vi "Read Value.vi"(6 "Gantry in":refnum<class "Gantry.lvclass">, 8 "error in (no error)":errorcluster, 10 "String in":string, 11 "gScript Interpreter in":refnum<class "gScript Interpreter.lvclass">) -> (0 "error out":errorcluster, 2 "Memory Cell":T1, 3 "gScript Interpreter out":refnum<class "gScript Interpreter.lvclass">, 4 "Gantry out":refnum<class "Gantry.lvclass">)   [LabVIEW 2026, in "gScript Interpreter.lvclass"]
uses:
  gScript Interpreter.lvclass
  Type Definitions/Memory Cell.ctl
  Type Definitions/Memory Cell Type Enum.ctl
  Shared Components/Gantry Class/Gantry.lvclass
  <vilib>/ErrorRing/Error Ring.xnode
  <vilib>/regexp/Match Regular Expression.xnode
  Shared Components/FlexWorktable/FlexWorktable.lvclass
  gScript Interpreter.lvclass/gScript Interpreter.ctl
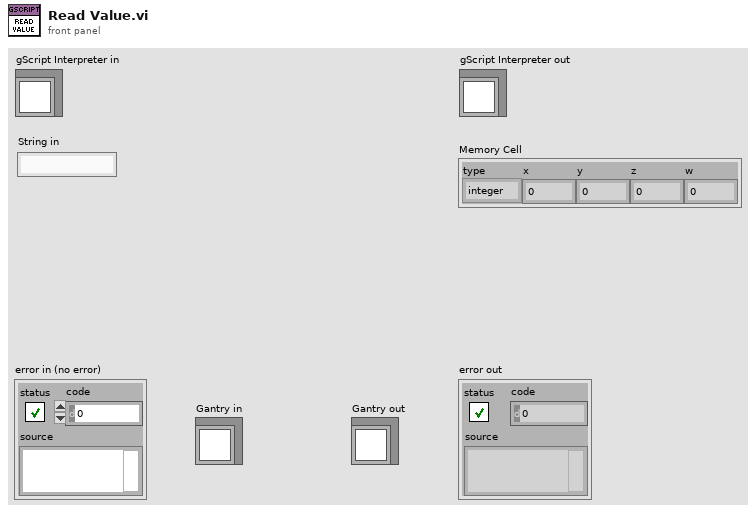
[diagram p1: front panel]
types:
  T1 = typedef "Memory Cell.ctl" = cluster{"type":T2, "x":dbl, "y":dbl, "z":dbl, "w":dbl}
  T2 = typedef "Memory Cell Type Enum.ctl" = enum16{"integer", "float", "vector", "rotation"}
  T3 = cluster{i32, dbl, string, bool, "Orient3d Class.lvclass":refnum<class "Orient3d.lvclass">, "Vec3d Class.lvclass":refnum<class "Vec3d.lvclass">}
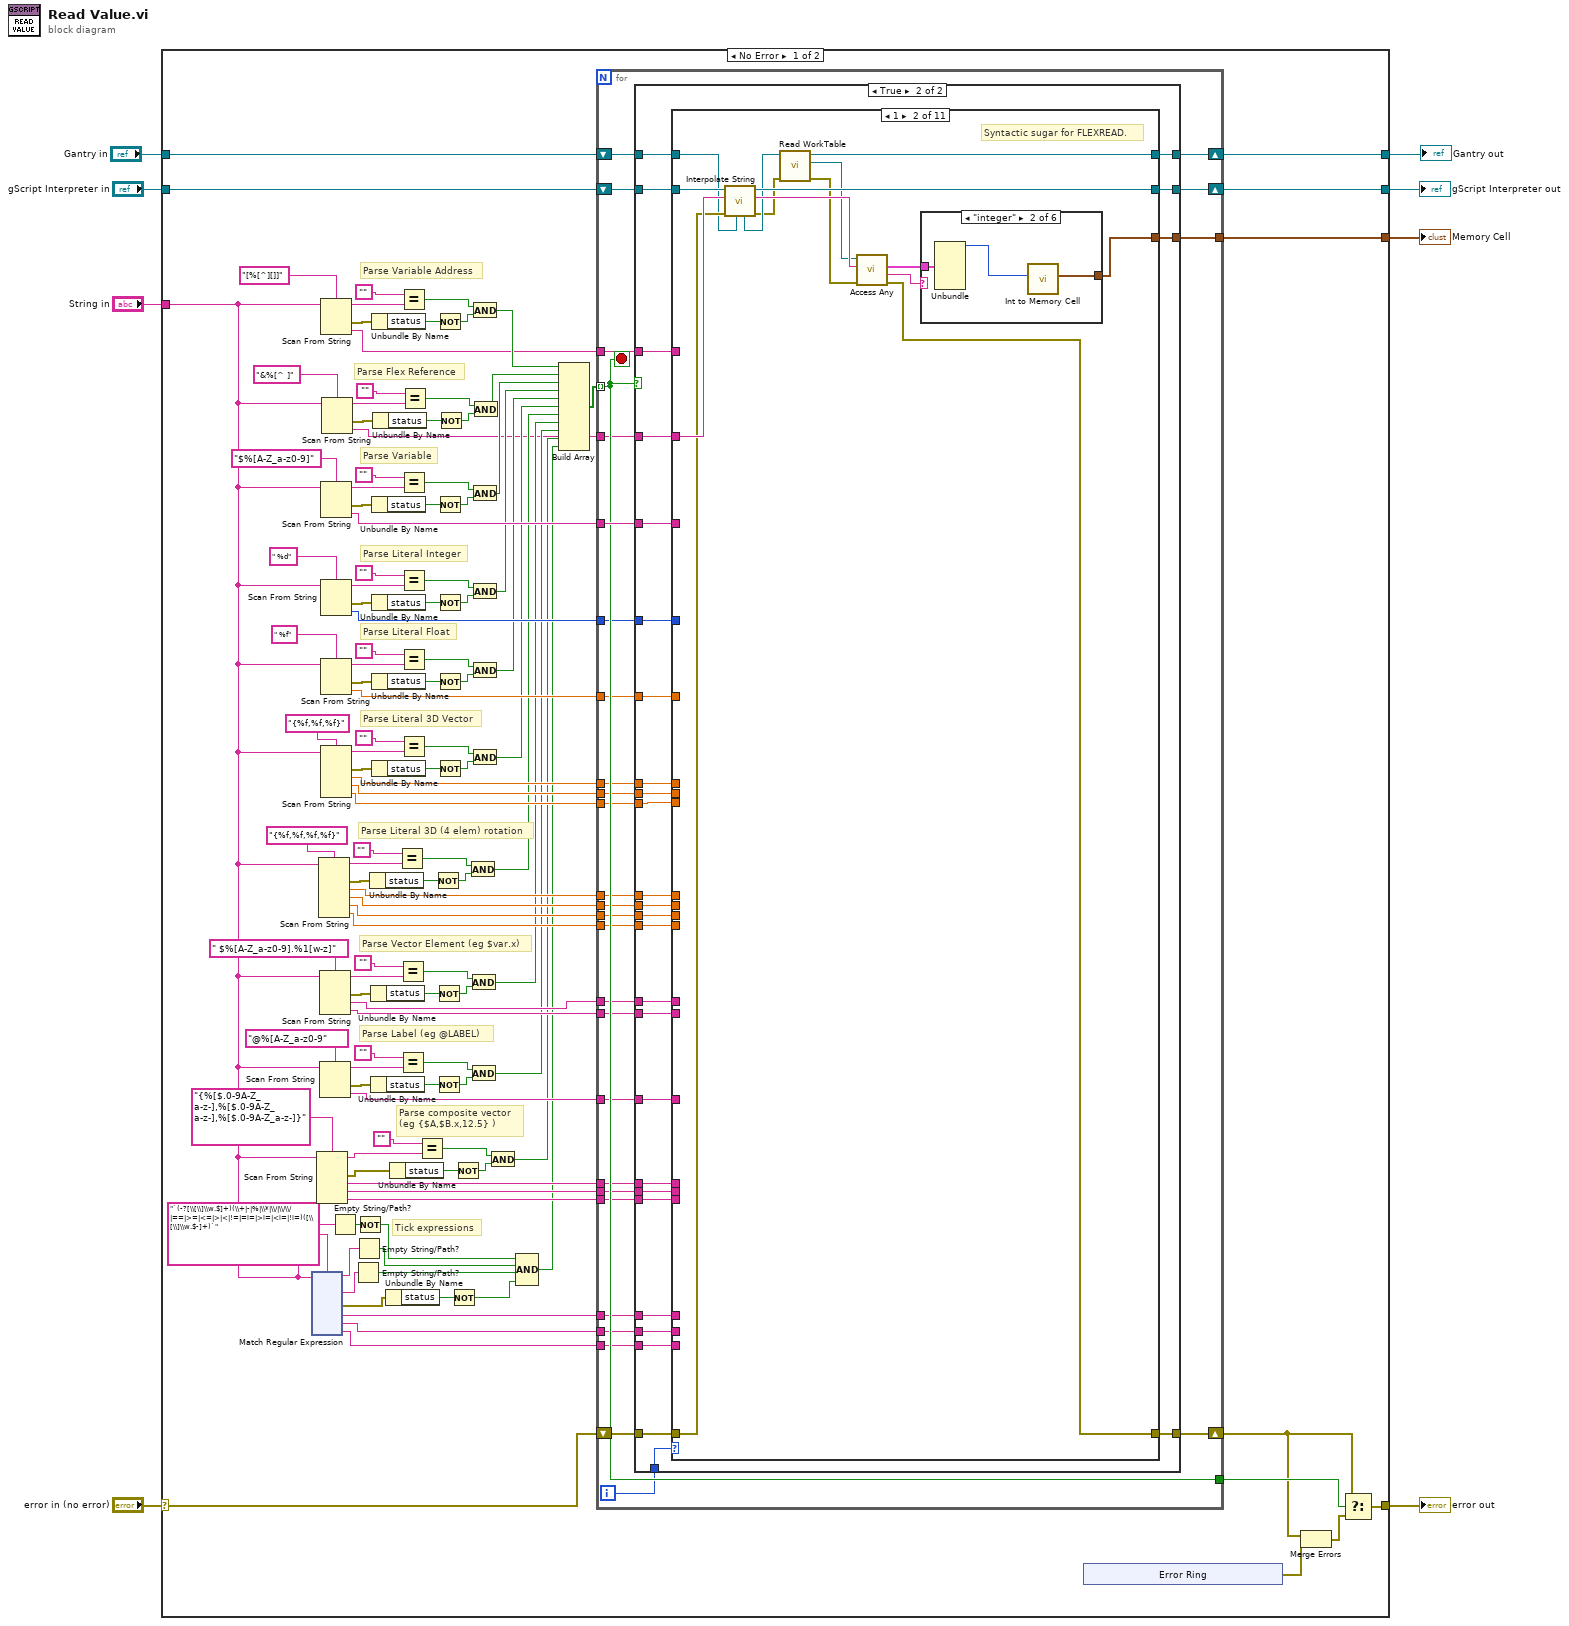
[diagram p0: block diagram]
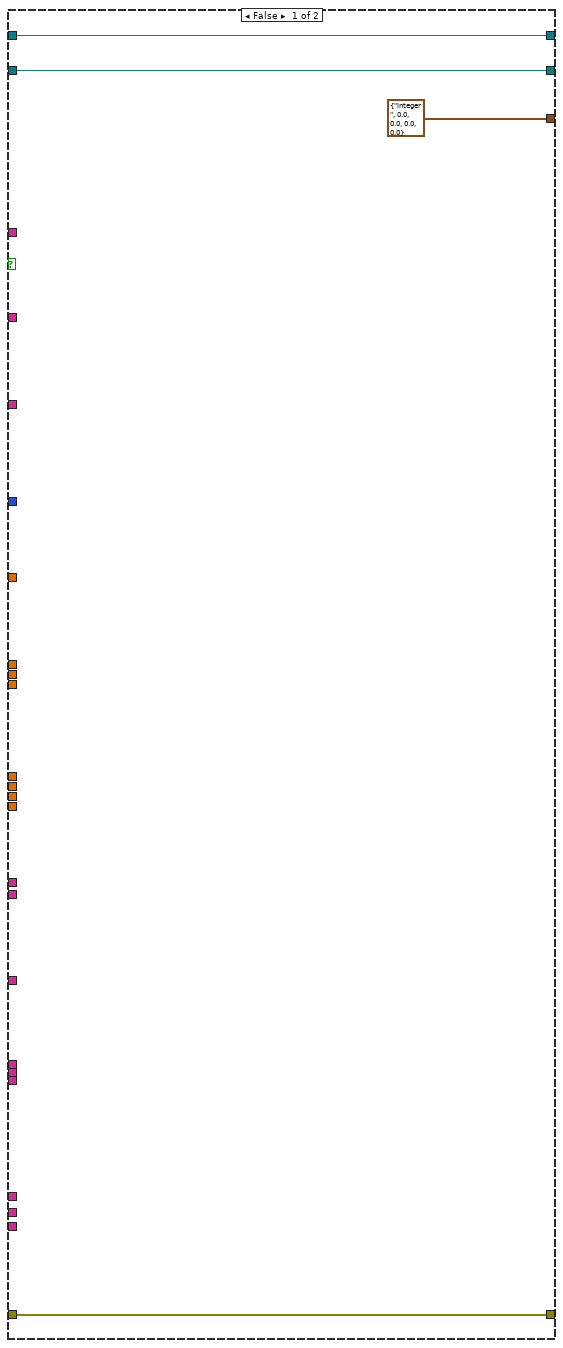
[diagram p2: hidden frame]
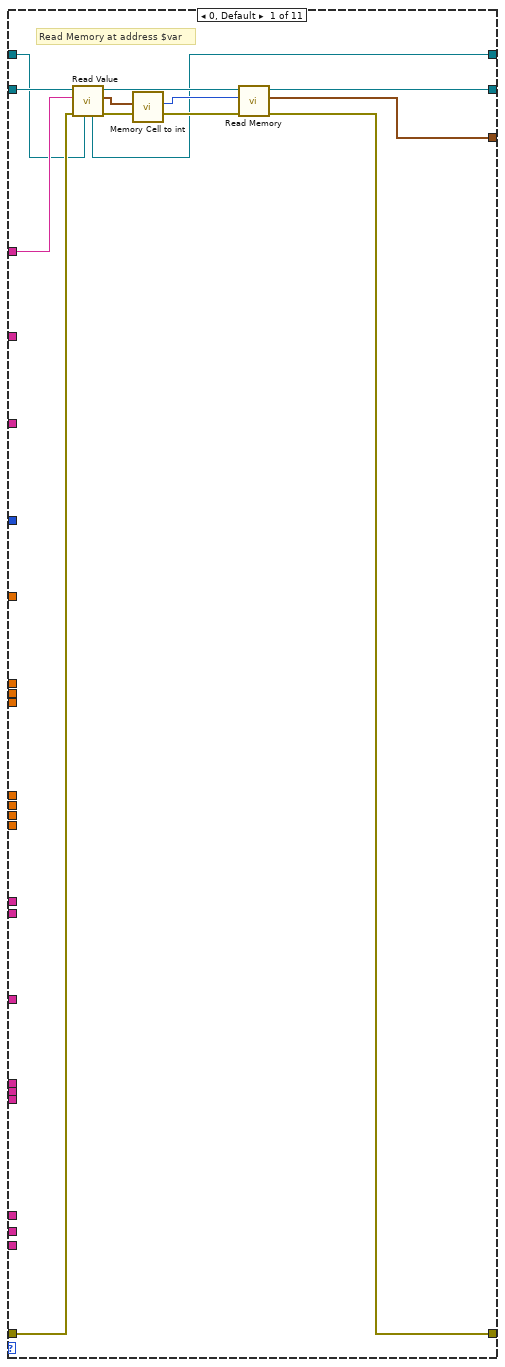
[diagram p3: hidden frame]
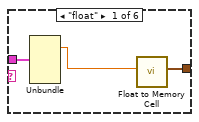
[diagram p4: hidden frame]
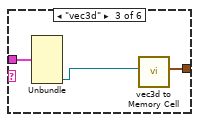
[diagram p5: hidden frame]
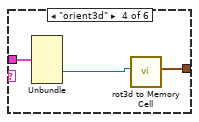
[diagram p6: hidden frame]
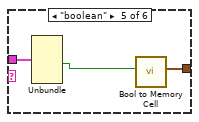
[diagram p7: hidden frame]
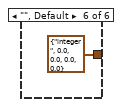
[diagram p8: hidden frame]
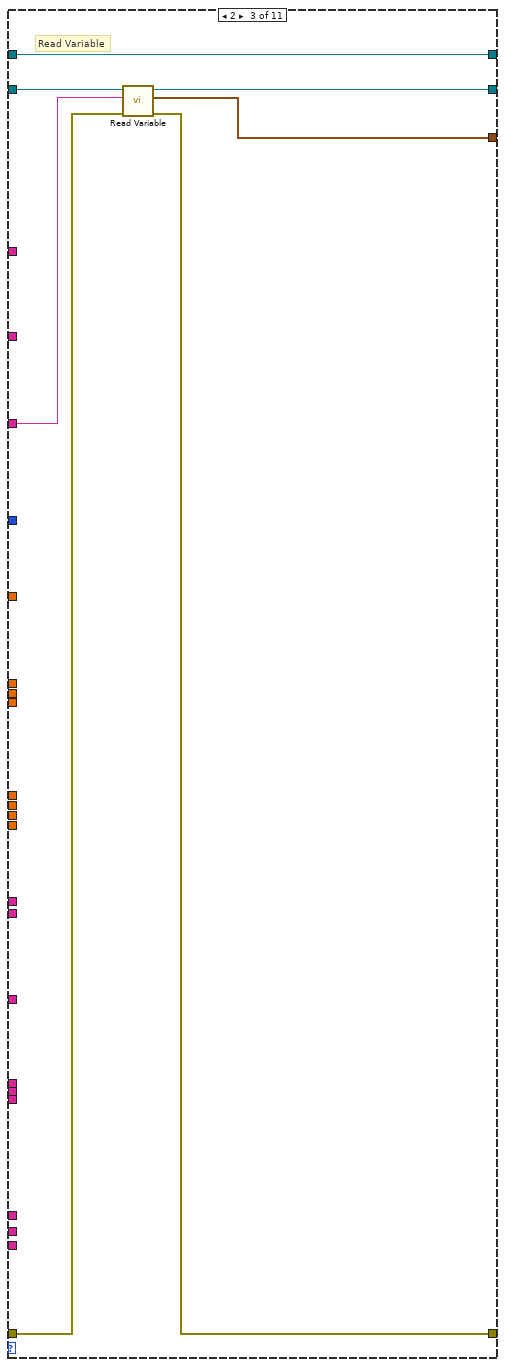
[diagram p9: hidden frame]
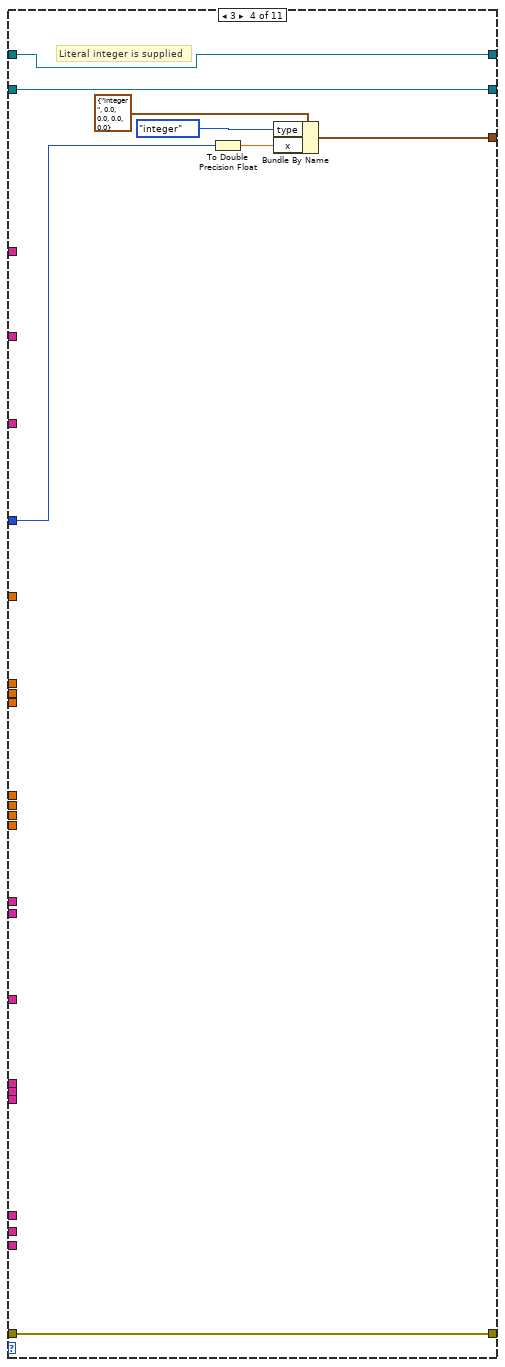
[diagram p10: hidden frame]
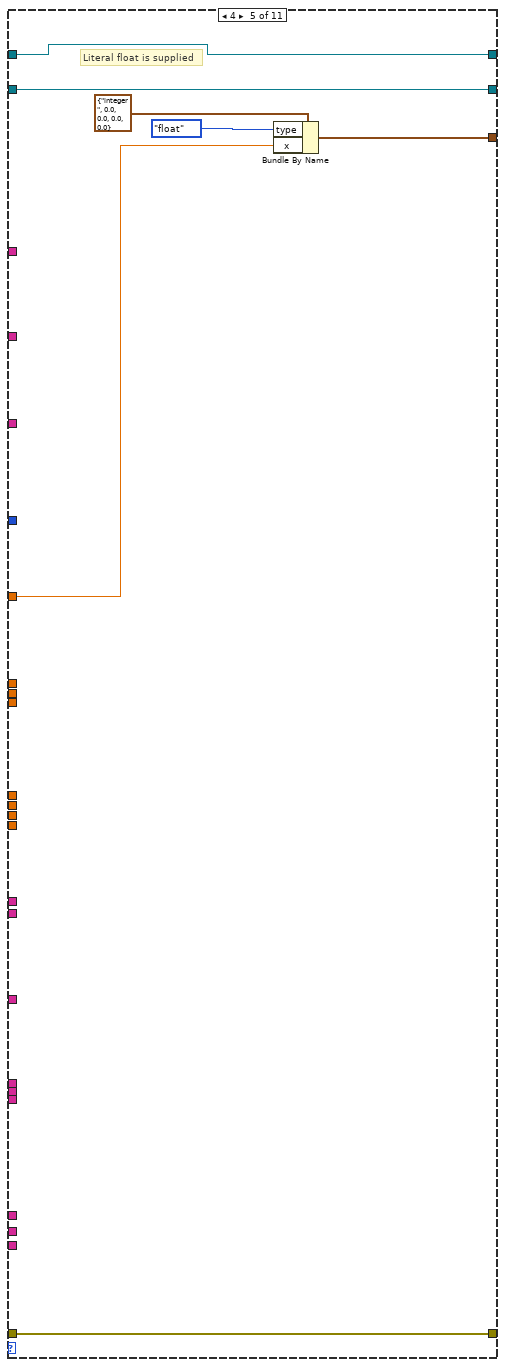
[diagram p11: hidden frame]
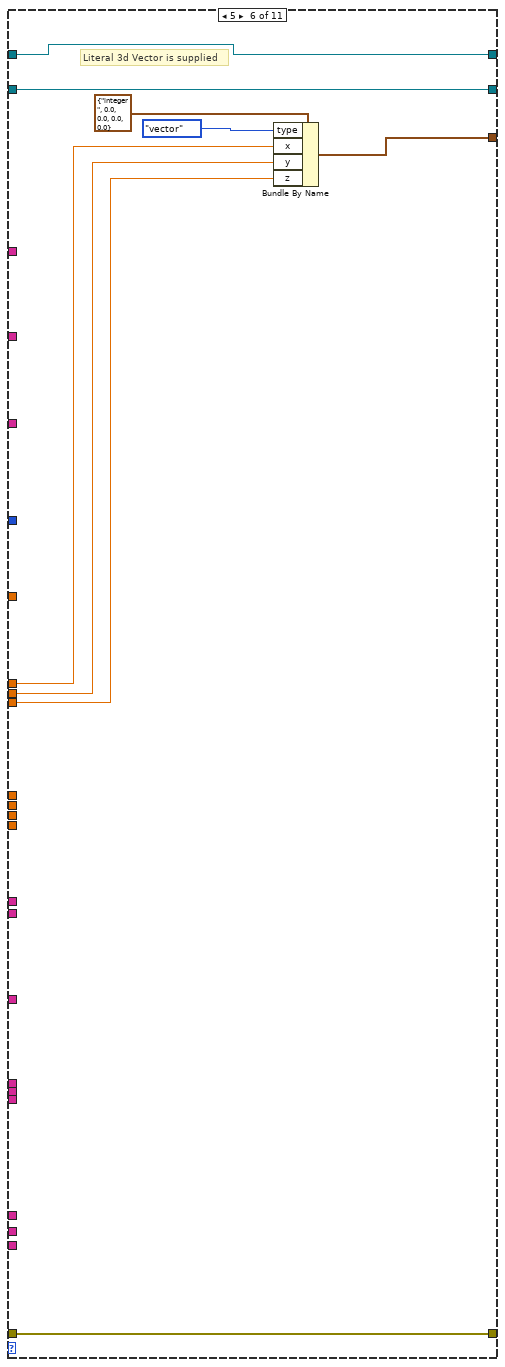
[diagram p12: hidden frame]
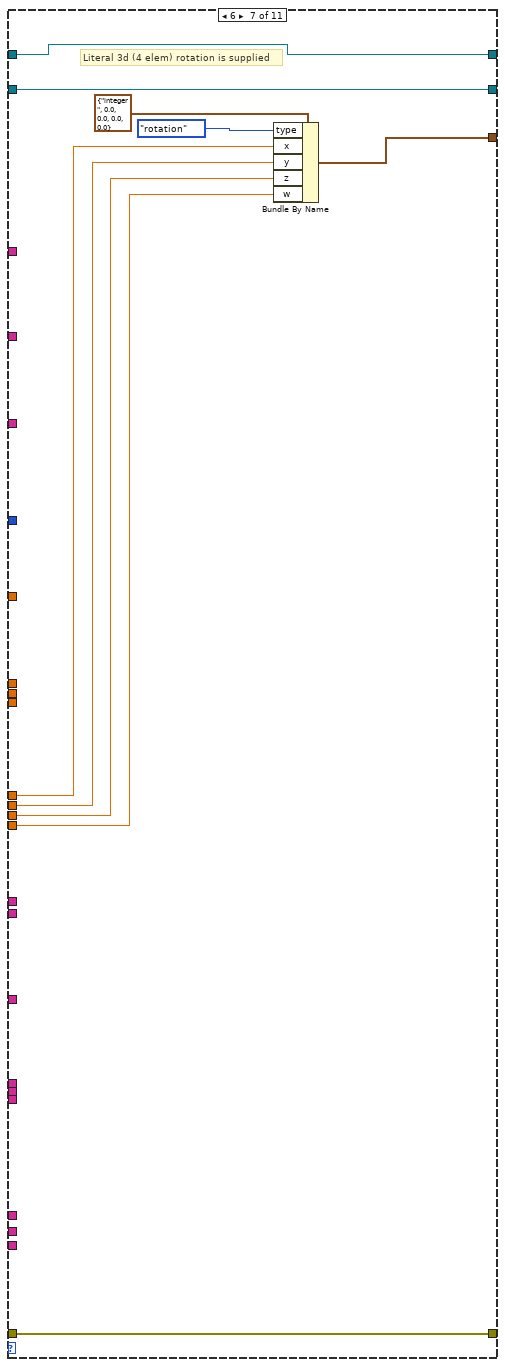
[diagram p13: hidden frame]
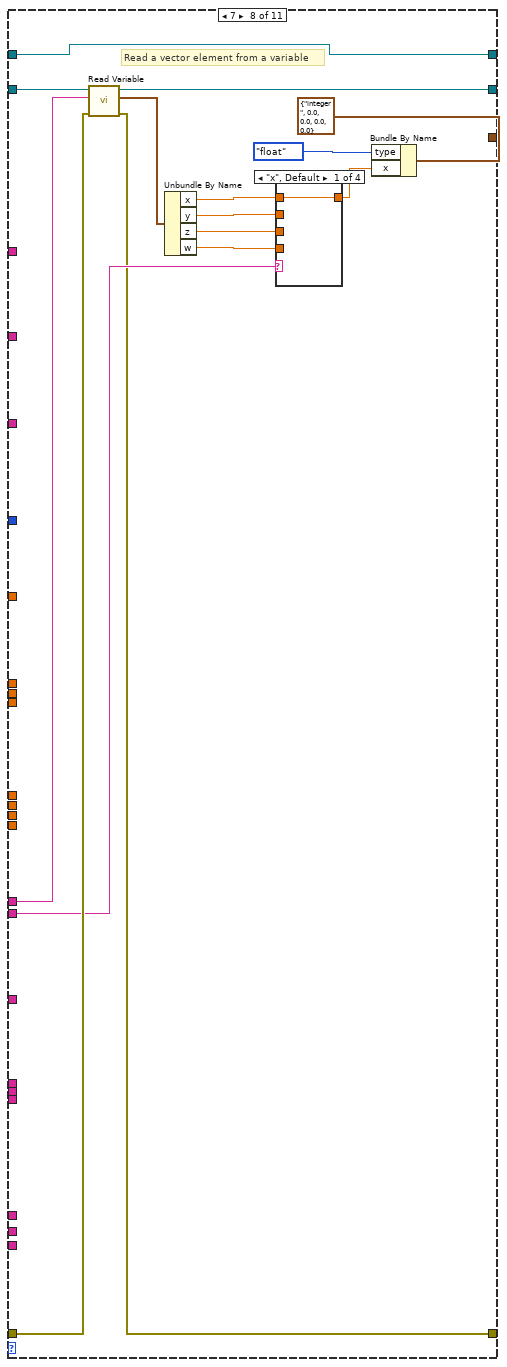
[diagram p14: hidden frame]
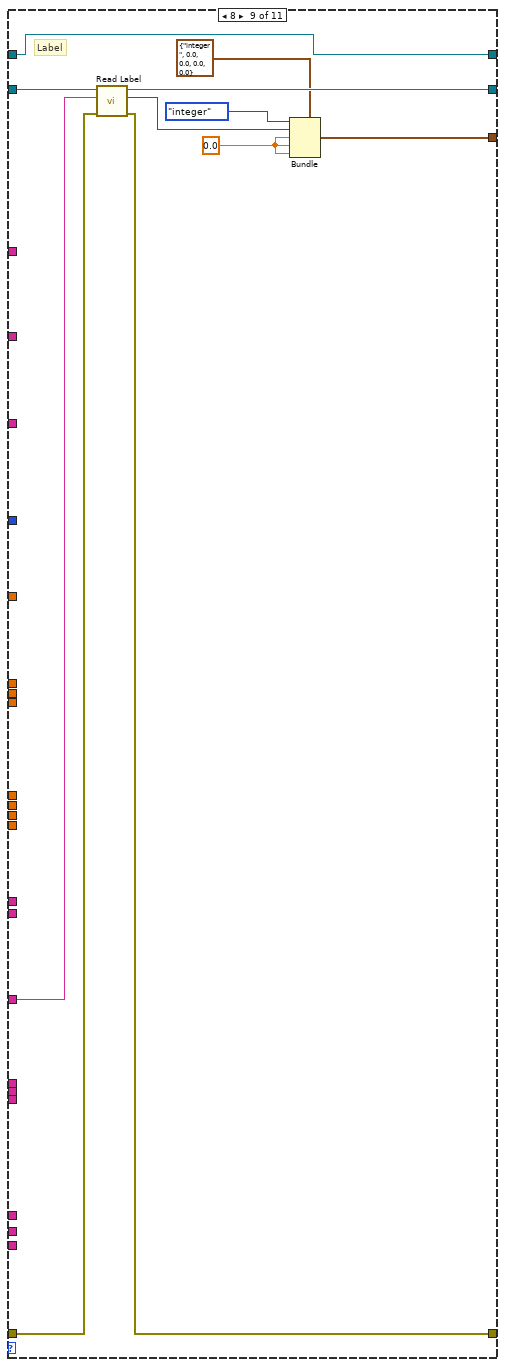
[diagram p18: hidden frame]
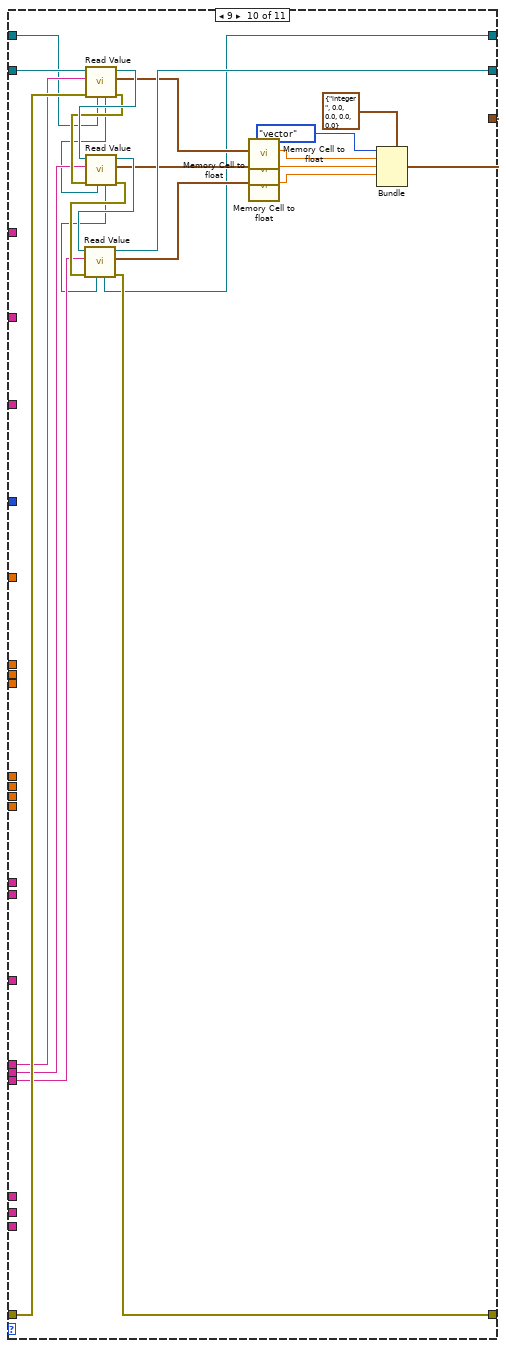
[diagram p19: hidden frame]
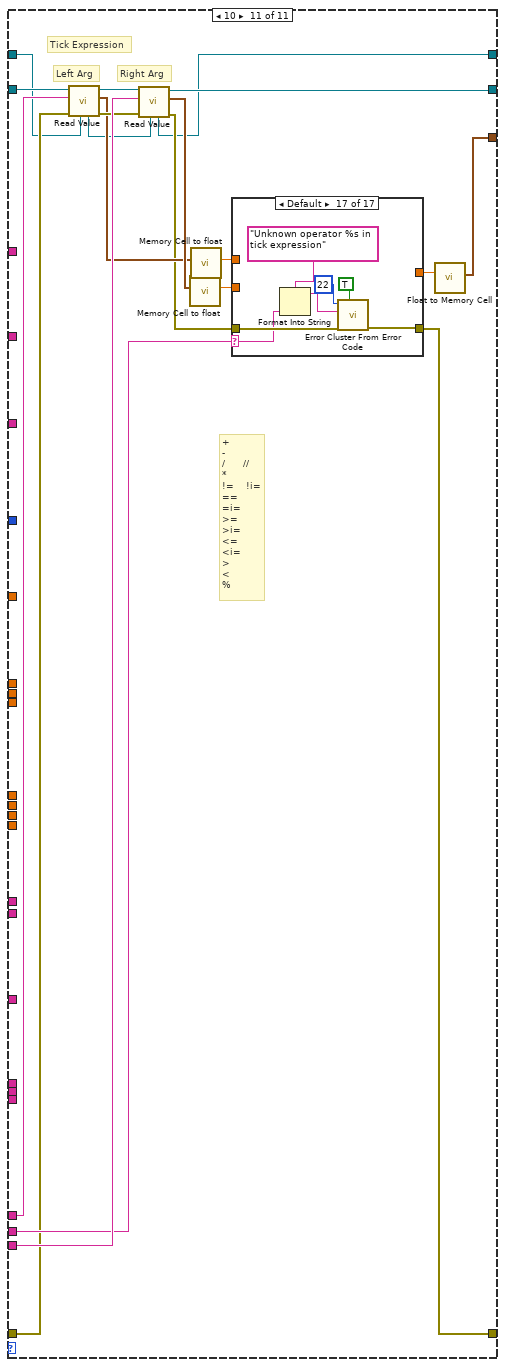
[diagram p20: hidden frame]
diagram:
  n1 = case shown="No Error" "error in (no error)" {
    selector: "error in (no error)" -> [w112 w581]
    tunnel: [w68 w581] -> w7
    tunnel: [w113 w580] -> w5
    tunnel: "gScript Interpreter in" -> [w114 w580]
    tunnel: "String in" -> [w11 _]
    tunnel: [w111 _] -> w3
    tunnel: "Gantry in" -> [w10 w579]
    tunnel: [w9 w579] -> w1
    frame No Error {
      # "Parse Flex Reference"
      # "Tick expressions"
      # "Parse composite vector\n(eg {$A,$B.x,12.5} )"
      # "Parse Label (eg @LABEL)"
      # "Parse Literal 3D (4 elem) rotation"
      # "Parse Literal 3D Vector"
      # "Parse Vector Element (eg $var.x)"
      # "Parse Literal Float"
      # "Parse Literal Integer"
      # "Parse Variable"
      # "Parse Variable Address"
      n2 = xnode "Match Regular Expression"("input string"=w11, "regular expression"="`(-?[\\[\\]\\w.$]+)(\\+|-|%|\\*|\\/|\\/\\/|==|>=|<=|>|<|!=|=i=|>i=|<i=|!i=)([\\[\\]\\w.$-]+)`") -> ("before match"=w28:string, "after match"=w27:string, "error out"=w33:errorcluster, "submatch 1"=w31:string, "submatch 2"=w30:string, "submatch 3"=w29:string)  [unwired: 4 in, 2 out]
      n3 = Scan From String(format string="{%[$.0-9A-Z_a-z-],%[$.0-9A-Z_a-z-],%[$.0-9A-Z_a-z-]}", input string=w11) -> (remaining string=w37:string, error out=w36:errorcluster, output 1=w44:string, output 2=w43:string, output 3=w42:string)  [unwired: 5 in, 1 out]
      n4 = Scan From String(format string="{%f,%f,%f,%f}", input string=w11) -> (remaining string=w66:string, error out=w64:errorcluster, output 1=w59:dbl, output 2=w58:dbl, output 3=w56:dbl, output 4=w57:dbl)  [unwired: 6 in, 1 out]
      n5 = Scan From String(format string=" $%[A-Z_a-z0-9].%1[w-z]", input string=w11) -> (remaining string=w91:string, error out=w89:errorcluster, output 1=w85:string, output 2=w84:string)  [unwired: 4 in, 1 out]
      n6 = Scan From String(format string="@%[A-Z_a-z0-9", input string=w11) -> (remaining string=w53:string, error out=w51:errorcluster, output 1=w46:string)  [unwired: 3 in, 1 out]
      n7 = Scan From String(format string="[%[^][]]", input string=w11) -> (remaining string=w132:string, error out=w130:errorcluster, output 1=w117:string)  [unwired: 3 in, 1 out]
      n8 = Scan From String(format string="$%[A-Z_a-z0-9]", input string=w11) -> (remaining string=w125:string, error out=w123:errorcluster, output 1=w115:string)  [unwired: 3 in, 1 out]
      n9 = Scan From String(format string=" %d", input string=w11) -> (remaining string=w109:string, error out=w107:errorcluster, output 1=w103:i32)  [unwired: 3 in, 1 out]
      n10 = Scan From String(format string=" %f", input string=w11) -> (remaining string=w100:string, error out=w98:errorcluster, output 1=w93:dbl)  [unwired: 3 in, 1 out]
      n11 = Scan From String(format string="{%f,%f,%f}", input string=w11) -> (remaining string=w82:string, error out=w80:errorcluster, output 1=w76:dbl, output 2=w75:dbl, output 3=w74:dbl)  [unwired: 5 in, 1 out]
      n12 = Scan From String(format string="&%[^ ]", input string=w11) -> (remaining string=w19:string, error out=w17:errorcluster, output 1=w13:string)  [unwired: 3 in, 1 out]
      n13 = Empty String/Path?(string/path=w11) -> (empty?=w24:bool)
      n14 = Empty String/Path?(string/path=w27) -> (empty?=w22:bool)
      n15 = Empty String/Path?(string/path=w28) -> (empty?=w23:bool)
      n16 = Not(x=w24) -> (.not. x?=w21:bool)
      n17 = Unbundle By Name(w64) -> ("status"=w62:bool)
      n18 = Unbundle By Name(w89) -> ("status"=w87:bool)
      n19 = Unbundle By Name(w51) -> ("status"=w49:bool)
      n20 = Unbundle By Name(w130) -> ("status"=w128:bool)
      n21 = Unbundle By Name(w123) -> ("status"=w121:bool)
      n22 = Unbundle By Name(w107) -> ("status"=w105:bool)
      n23 = Unbundle By Name(w98) -> ("status"=w96:bool)
      n24 = Unbundle By Name(w80) -> ("status"=w78:bool)
      n25 = Unbundle By Name(w17) -> ("status"=w15:bool)
      n26 = Unbundle By Name(w33) -> ("status"=w32:bool)
      n27 = Unbundle By Name(w36) -> ("status"=w39:bool)
      n28 = Equal?(x="", y=w66) -> (x = y?=w63:bool)
      n29 = Equal?(x="", y=w91) -> (x = y?=w88:bool)
      n30 = Equal?(x="", y=w53) -> (x = y?=w50:bool)
      n31 = Equal?(x="", y=w132) -> (x = y?=w129:bool)
      n32 = Equal?(x="", y=w125) -> (x = y?=w122:bool)
      n33 = Equal?(x="", y=w109) -> (x = y?=w106:bool)
      n34 = Equal?(x="", y=w100) -> (x = y?=w97:bool)
      n35 = Equal?(x="", y=w82) -> (x = y?=w79:bool)
      n36 = Equal?(x="", y=w19) -> (x = y?=w16:bool)
      n37 = Equal?(x="", y=w37) -> (x = y?=w40:bool)
      n38 = Not(x=w62) -> (.not. x?=w61:bool)
      n39 = Not(x=w87) -> (.not. x?=w86:bool)
      n40 = Not(x=w49) -> (.not. x?=w48:bool)
      n41 = Not(x=w128) -> (.not. x?=w127:bool)
      n42 = Not(x=w121) -> (.not. x?=w120:bool)
      n43 = Not(x=w105) -> (.not. x?=w104:bool)
      n44 = Not(x=w96) -> (.not. x?=w95:bool)
      n45 = Not(x=w78) -> (.not. x?=w77:bool)
      n46 = Not(x=w15) -> (.not. x?=w14:bool)
      n47 = Not(x=w32) -> (.not. x?=w26:bool)
      n48 = Not(x=w39) -> (.not. x?=w38:bool)
      n49 = And(x=w63, y=w61) -> (x .and. y?=w60:bool)
      n50 = And(x=w88, y=w86) -> (x .and. y?=w55:bool)
      n51 = And(x=w50, y=w48) -> (x .and. y?=w47:bool)
      n52 = And(x=w129, y=w127) -> (x .and. y?=w119:bool)
      n53 = And(x=w122, y=w120) -> (x .and. y?=w118:bool)
      n54 = And(x=w106, y=w104) -> (x .and. y?=w102:bool)
      n55 = And(x=w97, y=w95) -> (x .and. y?=w94:bool)
      n56 = And(x=w79, y=w77) -> (x .and. y?=w73:bool)
      n57 = And(x=w16, y=w14) -> (x .and. y?=w12:bool)
      n58 = And(x=w40, y=w38) -> (x .and. y?=w35:bool)
      n59 = Compound Arithmetic op=AND(w21, w23, w22, w26) -> (w25:bool)
      n60 = Build Array(w119, w12, w118, w102, w94, w73, w60, w55, w47, w35, w25) -> (w116:bool[])
      n61 = for {
        tunnel: w117 -> [w288]
        tunnel: w116 -> [w284] mode=indexing
        tunnel: w115 -> [w287]
        shift-right: [w285] -> w113
        shift-left: w114 -> [w286]
        tunnel: [w284] -> w72
        tunnel: [w282] -> w111
        shift-right: [w280] -> w70
        shift-left: w112 -> [w281]
        tunnel: w103 -> [w279]
        tunnel: w93 -> [w278]
        tunnel: w85 -> [w277]
        tunnel: w84 -> [w276]
        tunnel: w76 -> [w275]
        tunnel: w75 -> [w274]
        tunnel: w74 -> [w273]
        tunnel: w59 -> [w272]
        tunnel: w58 -> [w271]
        tunnel: w56 -> [w270]
        tunnel: w57 -> [w269]
        tunnel: w46 -> [w268]
        tunnel: w44 -> [w267]
        tunnel: w43 -> [w266]
        tunnel: w42 -> [w265]
        tunnel: w31 -> [w264]
        tunnel: w30 -> [w263]
        tunnel: w29 -> [w262]
        tunnel: w13 -> [w261]
        shift-right: [w259] -> w9
        shift-left: w10 -> [w260]
        i -> [w283]
        stop <- w284 stop-if-true
        n62 = case shown="True" w284 {
          tunnel: w288 -> [_ w321]
          tunnel: w287 -> [_ w320]
          tunnel: w286 -> [w292 w319]
          tunnel: [w292 w318] -> w285
          tunnel: w283 -> [_ w317]
          tunnel: [T1 {"type"=enum."integer", "x"=0.0, "y"=0.0, "z"=0.0, "w"=0.0} ("Memory Cell") w316] -> w282
          tunnel: w281 -> [w290 w315]
          tunnel: [w290 w314] -> w280
          tunnel: w279 -> [_ w313]
          tunnel: w278 -> [_ w312]
          tunnel: w277 -> [_ w311]
          tunnel: w276 -> [_ w310]
          tunnel: w275 -> [_ w309]
          tunnel: w274 -> [_ w308]
          tunnel: w273 -> [_ w307]
          tunnel: w272 -> [_ w306]
          tunnel: w271 -> [_ w305]
          tunnel: w270 -> [_ w304]
          tunnel: w269 -> [_ w303]
          tunnel: w268 -> [_ w302]
          tunnel: w267 -> [_ w301]
          tunnel: w266 -> [_ w300]
          tunnel: w265 -> [_ w299]
          tunnel: w264 -> [_ w298]
          tunnel: w263 -> [_ w297]
          tunnel: w262 -> [_ w296]
          tunnel: w261 -> [_ w295]
          tunnel: w260 -> [w289 w294]
          tunnel: [w289 w293] -> w259
          frame False {
          }
          frame True {
            n63 = case shown="1" w317 {
              tunnel: w321 -> [w324 _ _ _ _ _ _ _ _ _ _]
              tunnel: w320 -> [_ _ w369 _ _ _ _ _ _ _ _]
              tunnel: w319 -> [w329 w347 w371 w379 w386 w395 w405 w418 w436 w460 w479]
              tunnel: [w332 w344 w368 w379 w386 w395 w405 w417 w435 w457 w475] -> w318
              tunnel: [w331 w342 w367 w377 w384 w393 w403 w420 w428 w448 w465] -> w316
              tunnel: w315 -> [w325 w340 w370 w373 w382 w391 w401 w416 w432 w456 w474]
              tunnel: [w330 w341 w366 w373 w382 w391 w401 w407 w429 w447 w464] -> w314
              tunnel: w313 -> [_ _ _ w374 _ _ _ _ _ _ _]
              tunnel: w312 -> [_ _ _ _ w381 _ _ _ _ _ _]
              tunnel: w311 -> [_ _ _ _ _ _ _ w415 _ _ _]
              tunnel: w310 -> [_ _ _ _ _ _ _ w414 _ _ _]
              tunnel: w309 -> [_ _ _ _ _ w390 _ _ _ _ _]
              tunnel: w308 -> [_ _ _ _ _ w389 _ _ _ _ _]
              tunnel: w307 -> [_ _ _ _ _ w388 _ _ _ _ _]
              tunnel: w306 -> [_ _ _ _ _ _ w400 _ _ _ _]
              tunnel: w305 -> [_ _ _ _ _ _ w399 _ _ _ _]
              tunnel: w304 -> [_ _ _ _ _ _ w398 _ _ _ _]
              tunnel: w303 -> [_ _ _ _ _ _ w397 _ _ _ _]
              tunnel: w302 -> [_ _ _ _ _ _ _ _ w430 _ _]
              tunnel: w301 -> [_ _ _ _ _ _ _ _ _ w453 _]
              tunnel: w300 -> [_ _ _ _ _ _ _ _ _ w452 _]
              tunnel: w299 -> [_ _ _ _ _ _ _ _ _ w451 _]
              tunnel: w298 -> [_ _ _ _ _ _ _ _ _ _ w478]
              tunnel: w297 -> [_ _ _ _ _ _ _ _ _ _ w476]
              tunnel: w296 -> [_ _ _ _ _ _ _ _ _ _ w477]
              tunnel: w295 -> [_ w348 _ _ _ _ _ _ _ _ _]
              tunnel: w294 -> [w323 w339 w365 w372 w380 w387 w396 w406 w426 w440 w463]
              tunnel: [w322 w334 w365 w372 w380 w387 w396 w406 w426 w437 w461] -> w293
              frame 0, Default {
                # "Read Memory at address $var"
                n64 = call-dynamic "Read Value.vi"("Gantry in"=w323, "error in (no error)"=w325, "String in"=w324, "gScript Interpreter in"=w329) -> ("error out"=w326:errorcluster, "Memory Cell"=w327:T1, "gScript Interpreter out"=w328:refnum<class "gScript Interpreter.lvclass">, "Gantry out"=w322:refnum<class "Gantry.lvclass">)  [unwired: 4 in]
                n65 = call "Memory Cell to int.vi"("Memory Cell"=w327) -> ("Int out"=w333:i32)  [unwired: 10 in]
                n66 = call-dynamic "Read Memory.vi"("error in (no error)"=w326, "Memory Address"=w333, "gScript Interpreter in"=w328) -> ("error out"=w330:errorcluster, "Memory Cell"=w331:T1, "gScript Interpreter out"=w332:refnum<class "gScript Interpreter.lvclass">)  [unwired: 6 in]
              }
              frame 1 {
                # "Syntactic sugar for FLEXREAD."
                n67 = call-dynamic "Interpolate String.vi"("Gantry in"=w339, "error in (no error)"=w340, "Input String"=w348, "gScript Interpreter in"=w347) -> ("error out"=w336:errorcluster, "Output String"=w343:string, "gScript Interpreter out"=w344:refnum<class "gScript Interpreter.lvclass">, "Gantry out"=w338:refnum<class "Gantry.lvclass">)  [unwired: 4 in]
                n68 = call-dynamic "Read WorkTable.vi"("error in"=w336, "Gantry Class in"=w338) -> ("error out"=w335:errorcluster, "Worktable"=w337:refnum<class "FlexWorktable.lvclass">, "Gantry Class out"=w334:refnum<class "Gantry.lvclass">)  [unwired: 7 in]
                n69 = call-dynamic "Access Any.vi"("error in (no error)"=w335, "Key"=w343, "FlexWorktable in"=w337) -> ("error out"=w341:errorcluster, "Type"=w345:string, "Items out"=w346:T3)  [unwired: 5 in, 1 out]
                n70 = case shown="\"integer\"" w345 {
                  tunnel: [w351 w354 w357 w360 w362 T1 {"type"=enum."integer", "x"=0.0, "y"=0.0, "z"=0.0, "w"=0.0} ("Memory Cell")] -> w342
                  tunnel: w346 -> [w350 w353 w356 w359 w363 _]
                  frame "float" {
                    n71 = Unbundle(w350) -> (w349:dbl)  [unwired: 5 out]
                    n72 = call "Float to Memory Cell.vi"("Float in"=w349) -> ("Memory Cell"=w351:T1)  [unwired: 10 in]
                  }
                  frame "integer" {
                    n73 = Unbundle(w353) -> (w352:i32)  [unwired: 5 out]
                    n74 = call "Int to Memory Cell.vi"("Numeric"=w352) -> ("Memory Cell"=w354:T1)  [unwired: 10 in]
                  }
                  frame "vec3d" {
                    n75 = Unbundle(w356) -> ("Vec3d Class.lvclass"=w355:refnum<class "Vec3d.lvclass">)  [unwired: 5 out]
                    n76 = call "vec3d to Memory Cell.vi"("Vec3d in"=w355) -> ("Memory Cell"=w357:T1)  [unwired: 10 in]
                  }
                  frame "orient3d" {
                    n77 = Unbundle(w359) -> ("Orient3d Class.lvclass"=w358:refnum<class "Orient3d.lvclass">)  [unwired: 5 out]
                    n78 = call "rot3d to Memory Cell.vi"("Orient3d in"=w358) -> ("Memory Cell"=w360:T1)  [unwired: 10 in]
                  }
                  frame "boolean" {
                    n79 = Unbundle(w363) -> (w361:bool)  [unwired: 5 out]
                    n80 = call "Bool to Memory Cell.vi"("Boolean in"=w361) -> ("Memory Cell"=w362:T1)  [unwired: 10 in]
                  }
                  frame "", Default {
                  }
                }
              }
              frame 2 {
                # "Read Variable"
                n81 = call-dynamic "Read Variable.vi"("error in (no error)"=w370, "Variable Name"=w369, "gScript Interpreter in"=w371) -> ("error out"=w366:errorcluster, "Memory Cell"=w367:T1, "gScript Interpreter out"=w368:refnum<class "gScript Interpreter.lvclass">)  [unwired: 6 in]
              }
              frame 3 {
                # "Literal integer is supplied"
                n82 = To Double Precision Float(number=w374) -> (double precision float=w375:dbl)
                n83 = Bundle By Name(cluster=T1 {"type"=enum."integer", "x"=0.0, "y"=0.0, "z"=0.0, "w"=0.0} ("Memory Cell"), "type"=Memory_Cell_Type_Enum."integer", "x"=w375) -> (w377:T1)
              }
              frame 4 {
                # "Literal float is supplied"
                n84 = Bundle By Name(cluster=T1 {"type"=enum."integer", "x"=0.0, "y"=0.0, "z"=0.0, "w"=0.0} ("Memory Cell"), "type"=Memory_Cell_Type_Enum."float", "x"=w381) -> (w384:T1)
              }
              frame 5 {
                # "Literal 3d Vector is supplied"
                n85 = Bundle By Name(cluster=T1 {"type"=enum."integer", "x"=0.0, "y"=0.0, "z"=0.0, "w"=0.0} ("Memory Cell"), "type"=Memory_Cell_Type_Enum."vector", "x"=w390, "y"=w389, "z"=w388) -> (w393:T1)
              }
              frame 6 {
                # "Literal 3d (4 elem) rotation is supplied"
                n86 = Bundle By Name(cluster=T1 {"type"=enum."integer", "x"=0.0, "y"=0.0, "z"=0.0, "w"=0.0} ("Memory Cell"), "type"=Memory_Cell_Type_Enum."rotation", "x"=w400, "y"=w399, "z"=w398, "w"=w397) -> (w403:T1)
              }
              frame 7 {
                # "Read a vector element from a variable"
                n87 = call-dynamic "Read Variable.vi"("error in (no error)"=w416, "Variable Name"=w415, "gScript Interpreter in"=w418) -> ("error out"=w407:errorcluster, "Memory Cell"=w413:T1, "gScript Interpreter out"=w417:refnum<class "gScript Interpreter.lvclass">)  [unwired: 6 in]
                n88 = Unbundle By Name(w413) -> ("x"=w412:dbl, "y"=w411:dbl, "z"=w410:dbl, "w"=w409:dbl)
                n89 = case shown="\"x\", Default" w414 {
                  tunnel: w412 -> [w422 _ _ _]
                  tunnel: w411 -> [_ w423 _ _]
                  tunnel: w410 -> [_ _ w424 _]
                  tunnel: w409 -> [_ _ _ w425]
                  tunnel: [w422 w423 w424 w425] -> w408
                  frame "x", Default {
                  }
                  frame "y" {
                  }
                  frame "z" {
                  }
                  frame "w" {
                  }
                }
                n90 = Bundle By Name(cluster=T1 {"type"=enum."integer", "x"=0.0, "y"=0.0, "z"=0.0, "w"=0.0} ("Memory Cell"), "type"=Memory_Cell_Type_Enum."float", "x"=w408) -> (w420:T1)
              }
              frame 8 {
                w427 = 0.0 ("y")
                # "Label"
                n91 = call-dynamic "Read Label.vi"("error in (no error)"=w432, "Label"=w430, "gScript Interpreter in"=w436) -> ("error out"=w429:errorcluster, "Line"=w433:i32, "gScript Interpreter out"=w435:refnum<class "gScript Interpreter.lvclass">)  [unwired: 5 in, 1 out]
                n92 = Bundle(cluster=T1 {"type"=enum."integer", "x"=0.0, "y"=0.0, "z"=0.0, "w"=0.0} ("Memory Cell"), "type"=Memory_Cell_Type_Enum."integer", "x"=w433, "y"=w427, "z"=w427, "w"=w427) -> (w428:T1)
              }
              frame 9 {
                n93 = call-dynamic "Read Value.vi"("Gantry in"=w440, "error in (no error)"=w456, "String in"=w453, "gScript Interpreter in"=w460) -> ("error out"=w455:errorcluster, "Memory Cell"=w446:T1, "gScript Interpreter out"=w459:refnum<class "gScript Interpreter.lvclass">, "Gantry out"=w439:refnum<class "Gantry.lvclass">)  [unwired: 4 in]
                n94 = call-dynamic "Read Value.vi"("Gantry in"=w439, "error in (no error)"=w455, "String in"=w452, "gScript Interpreter in"=w459) -> ("error out"=w454:errorcluster, "Memory Cell"=w444:T1, "gScript Interpreter out"=w458:refnum<class "gScript Interpreter.lvclass">, "Gantry out"=w438:refnum<class "Gantry.lvclass">)  [unwired: 4 in]
                n95 = call-dynamic "Read Value.vi"("Gantry in"=w438, "error in (no error)"=w454, "String in"=w451, "gScript Interpreter in"=w458) -> ("error out"=w447:errorcluster, "Memory Cell"=w443:T1, "gScript Interpreter out"=w457:refnum<class "gScript Interpreter.lvclass">, "Gantry out"=w437:refnum<class "Gantry.lvclass">)  [unwired: 4 in]
                n96 = call "Memory Cell to float.vi"("Memory Cell"=w446) -> ("float out"=w445:dbl)  [unwired: 10 in]
                n97 = call "Memory Cell to float.vi"("Memory Cell"=w444) -> ("float out"=w442:dbl)  [unwired: 10 in]
                n98 = call "Memory Cell to float.vi"("Memory Cell"=w443) -> ("float out"=w441:dbl)  [unwired: 10 in]
                n99 = Bundle(cluster=T1 {"type"=enum."integer", "x"=0.0, "y"=0.0, "z"=0.0, "w"=0.0} ("Memory Cell"), "type"=Memory_Cell_Type_Enum."vector", "x"=w445, "y"=w442, "z"=w441) -> (w448:T1)  [unwired: 1 in]
              }
              frame 10 {
                # "+\n-\n/      //\n*\n!=    !i=\n==  =i=\n>=  >i=\n<=  <i=\n> \n<\n%"
                # "Right Arg"
                # "Left Arg"
                # "Tick Expression"
                n100 = call-dynamic "Read Value.vi"("Gantry in"=w463, "error in (no error)"=w474, "String in"=w478, "gScript Interpreter in"=w479) -> ("error out"=w473:errorcluster, "Memory Cell"=w470:T1, "gScript Interpreter out"=w472:refnum<class "gScript Interpreter.lvclass">, "Gantry out"=w462:refnum<class "Gantry.lvclass">)  [unwired: 4 in]
                n101 = call-dynamic "Read Value.vi"("Gantry in"=w462, "error in (no error)"=w473, "String in"=w477, "gScript Interpreter in"=w472) -> ("error out"=w467:errorcluster, "Memory Cell"=w471:T1, "gScript Interpreter out"=w475:refnum<class "gScript Interpreter.lvclass">, "Gantry out"=w461:refnum<class "Gantry.lvclass">)  [unwired: 4 in]
                n102 = call "Memory Cell to float.vi"("Memory Cell"=w471) -> ("float out"=w468:dbl)  [unwired: 10 in]
                n103 = call "Memory Cell to float.vi"("Memory Cell"=w470) -> ("float out"=w469:dbl)  [unwired: 10 in]
                n104 = case shown="Default" w476 {
                  selector: w476 -> [_ _ _ _ _ _ _ _ _ _ _ _ _ _ _ _ w575]
                  tunnel: w469 -> [w483 w487 w491 w495 w499 w503 w509 w515 w520 w528 w536 w544 w551 w557 w563 w569 _]
                  tunnel: w468 -> [w482 w486 w490 w494 w498 w502 w508 w514 w519 w527 w535 w543 w550 w556 w562 w568 _]
                  tunnel: w467 -> [w480 w484 w488 w492 w496 w500 w504 w510 w516 w524 w532 w540 w548 w554 w560 w566 w578]
                  tunnel: [w481 w485 w489 w493 w497 w501 w505 w511 w521 w529 w537 w545 w549 w555 w561 w567 _] -> w466
                  tunnel: [w480 w484 w488 w492 w496 w500 w504 w510 w516 w524 w532 w540 w548 w554 w560 w566 w577] -> w464
                  frame "+" {
                    n105 = Add(x=w483, y=w482) -> (x+y=w481:dbl)
                  }
                  frame "-" {
                    n106 = Subtract(x=w487, y=w486) -> (x-y=w485:dbl)
                  }
                  frame "%" {
                    n107 = Quotient & Remainder(x=w491, y=w490) -> (x-y*floor(x/y)=w489:dbl)  [unwired: 1 out]
                  }
                  frame "*" {
                    n108 = Multiply(x=w495, y=w494) -> (x*y=w493:dbl)
                  }
                  frame "/" {
                    n109 = Divide(x=w499, y=w498) -> (x/y=w497:dbl)
                  }
                  frame "//" {
                    n110 = Quotient & Remainder(x=w503, y=w502) -> (floor(x/y)=w501:dbl)  [unwired: 1 out]
                  }
                  frame "==" {
                    n111 = Equal?(x=w509, y=w508) -> (x = y?=w507:bool)
                    n112 = Boolean To (0,1)(Boolean=w507) -> (0, 1=w506:i16)
                    n113 = To Double Precision Float(number=w506) -> (double precision float=w505:dbl)
                  }
                  frame "!=" {
                    n114 = Not Equal?(x=w515, y=w514) -> (x != y?=w513:bool)
                    n115 = Boolean To (0,1)(Boolean=w513) -> (0, 1=w512:i16)
                    n116 = To Double Precision Float(number=w512) -> (double precision float=w511:dbl)
                  }
                  frame "=i=" {
                    n117 = To Long Integer(number=w520) -> (32bit integer=w517:i32)
                    n118 = To Long Integer(number=w519) -> (32bit integer=w518:i32)
                    n119 = Equal?(x=w517, y=w518) -> (x = y?=w523:bool)
                    n120 = Boolean To (0,1)(Boolean=w523) -> (0, 1=w522:i16)
                    n121 = To Double Precision Float(number=w522) -> (double precision float=w521:dbl)
                  }
                  frame ">i=" {
                    n122 = To Long Integer(number=w528) -> (32bit integer=w525:i32)
                    n123 = To Long Integer(number=w527) -> (32bit integer=w526:i32)
                    n124 = Greater Or Equal?(x=w525, y=w526) -> (x >= y?=w531:bool)
                    n125 = Boolean To (0,1)(Boolean=w531) -> (0, 1=w530:i16)
                    n126 = To Double Precision Float(number=w530) -> (double precision float=w529:dbl)
                  }
                  frame "<i=" {
                    n127 = To Long Integer(number=w536) -> (32bit integer=w533:i32)
                    n128 = To Long Integer(number=w535) -> (32bit integer=w534:i32)
                    n129 = Less Or Equal?(x=w533, y=w534) -> (x <= y?=w539:bool)
                    n130 = Boolean To (0,1)(Boolean=w539) -> (0, 1=w538:i16)
                    n131 = To Double Precision Float(number=w538) -> (double precision float=w537:dbl)
                  }
                  frame "!i=" {
                    n132 = To Long Integer(number=w544) -> (32bit integer=w541:i32)
                    n133 = To Long Integer(number=w543) -> (32bit integer=w542:i32)
                    n134 = Not Equal?(x=w541, y=w542) -> (x != y?=w547:bool)
                    n135 = Boolean To (0,1)(Boolean=w547) -> (0, 1=w546:i16)
                    n136 = To Double Precision Float(number=w546) -> (double precision float=w545:dbl)
                  }
                  frame ">=" {
                    n137 = Greater Or Equal?(x=w551, y=w550) -> (x >= y?=w552:bool)
                    n138 = Boolean To (0,1)(Boolean=w552) -> (0, 1=w553:i16)
                    n139 = To Double Precision Float(number=w553) -> (double precision float=w549:dbl)
                  }
                  frame "<=" {
                    n140 = Less Or Equal?(x=w557, y=w556) -> (x <= y?=w558:bool)
                    n141 = Boolean To (0,1)(Boolean=w558) -> (0, 1=w559:i16)
                    n142 = To Double Precision Float(number=w559) -> (double precision float=w555:dbl)
                  }
                  frame ">" {
                    n143 = Greater?(x=w563, y=w562) -> (0:w564:bool)
                    n144 = Boolean To (0,1)(Boolean=w564) -> (0, 1=w565:i16)
                    n145 = To Double Precision Float(number=w565) -> (double precision float=w561:dbl)
                  }
                  frame "<" {
                    n146 = Less?(x=w569, y=w568) -> (x < y?=w570:bool)
                    n147 = Boolean To (0,1)(Boolean=w570) -> (0, 1=w571:i16)
                    n148 = To Double Precision Float(number=w571) -> (double precision float=w567:dbl)
                  }
                  frame Default {
                    n149 = Format Into String(format string="Unknown operator %s in tick expression", w575) -> (resulting string=w574:string)  [unwired: 2 in, 1 out]
                    n150 = call <vilib>:"Error Cluster From Error Code.vi"("show call chain? (False)"=TRUE, "error in (no error)"=w578, "error message (\"\")"=w574, "error code (0)"=22) -> ("error out"=w577:errorcluster)  [unwired: 5 in]
                  }
                }
                n151 = call "Float to Memory Cell.vi"("Float in"=w466) -> ("Memory Cell"=w465:T1)  [unwired: 10 in]
              }
            }
          }
        }
      }
      n152 = xnode "Error Ring"() -> ("error out"=w71:errorcluster)
      n153 = Merge Errors(w70, w71) -> (w69:errorcluster)
      n154 = Select(t=w70, s=w72, f=w69) -> (s? t:f=w68:errorcluster)
    }
    frame Error {
    }
  }
  "error out" <- w7
  "gScript Interpreter out" <- w5
  "Memory Cell" <- w3
  "Gantry out" <- w1
